vi "st deviation (median).vi"(0 "X":dbl[](array[numeric])) -> (1 "median":dbl, 2 "standard deviation":dbl, 3 "variance":dbl)   [LabVIEW 2009]
uses:
  <vilib>/Analysis/NI_AALBase.lvlib
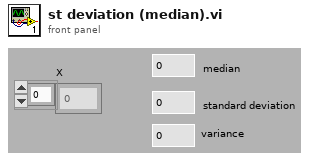
[diagram p1: front panel]
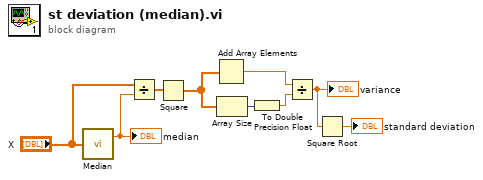
[diagram p0: block diagram]
diagram:
  n1 = call <vilib>:"Median.vi"("X"="X") -> ("median"=w1:dbl)  [unwired: 1 out]
  "median" <- w1
  n2 = Divide(x="X", y=w1) -> (x/y=w9:dbl[])
  n3 = Square(x=w9) -> (x^2=w7:dbl[])
  n4 = Add Array Elements(numeric array=w7) -> (sum=w6:dbl)
  n5 = Array Size(array=w7) -> (size(s)=w5:i32)
  n6 = To Double Precision Float(number=w5) -> (double precision float=w4:dbl)
  n7 = Divide(x=w6, y=w4) -> (x/y=w3:dbl)
  "variance" <- w3
  n8 = Square Root(x=w3) -> (sqrt(x)=→"standard deviation":dbl)
